vi "Instrument System Definition Example.vi"(10 "Instrument Addon Config Datalog Path":path, 11 "SysDef Path":path) -> (0 "error out":errorcluster)   [LabVIEW 2019]
uses:
  NationalInstruments.VeriStand.SystemDefinitionAPI
  Instrument System Definition API.lvlib
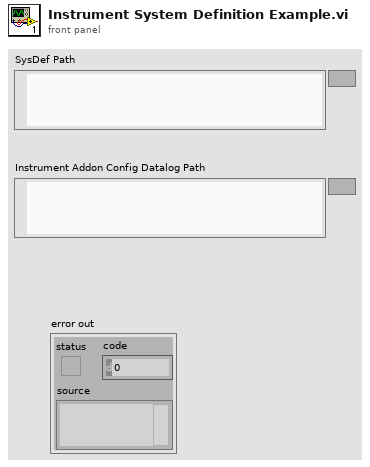
[diagram p1: front panel]
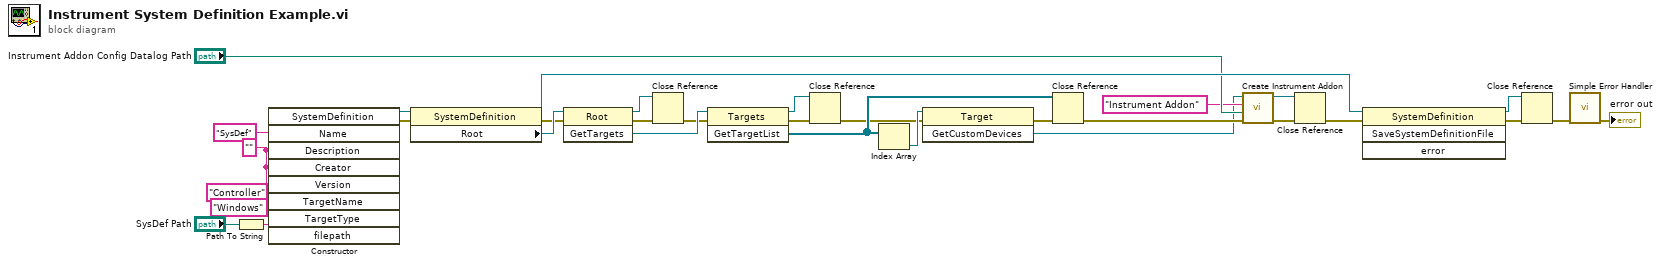
[diagram p0: block diagram]
diagram:
  w7 = "" ("Name")
  n1 = Path To String(path="SysDef Path") -> (string=w10:string)
  n2 = constructor class="SystemDefinition"("Name"="SysDef", "Description"=w7, "Creator"=w7, "Version"=w7, "TargetName"="Controller", "TargetType"="Windows", "filepath"=w10) -> (reference out=w32:refnum<k24>, error out=w28:errorcluster)  [unwired: 3 in, 8 out]
  n3 = property class="SystemDefinition"(reference=w32, error in=w28) -> (reference out=w26:refnum<k24>, error out=w27:errorcluster, "Root"=w31:refnum<k24>)
  n4 = invoke class="Root" method="GetTargets"(reference=w31, error in=w27) -> (reference out=w12:refnum<k24>, error out=w14:errorcluster, "GetTargets"=w30:refnum<k24>)  [unwired: 1 in]
  n5 = Close Reference(reference=w12, error in (no error)=w14) -> (error out=w13:errorcluster)
  n6 = invoke class="Targets" method="GetTargetList"(reference=w30, error in=w13) -> (reference out=w15:refnum<k24>, error out=w17:errorcluster, "GetTargetList"=w18:refnum<k24>[])  [unwired: 1 in]
  n7 = Close Reference(reference=w15, error in (no error)=w17) -> (error out=w16:errorcluster)
  n8 = Index Array(array=w18) -> (element=w29:refnum<k24>)  [unwired: 1 in]
  n9 = invoke class="Target" method="GetCustomDevices"(reference=w29, error in=w16) -> (error out=w20:errorcluster, "GetCustomDevices"=w3:refnum<k24>)  [unwired: 1 in, 1 out]
  n10 = Close Reference(reference=w18, error in (no error)=w20) -> (error out=w19:errorcluster)
  n11 = call "Create Instrument Addon.vi"("error in (no error)"=w19, "CD Config Path (.dat)"="Instrument Addon Config Datalog Path", "Name"="Instrument Addon", "Custom Devices Ref"=w3) -> ("error out"=w2:errorcluster, "Custom Devices Ref"=w21:refnum<k24>)  [unwired: 6 in]
  n12 = Close Reference(reference=w21, error in (no error)=w2) -> (error out=w22:errorcluster)
  n13 = invoke class="SystemDefinition" method="SaveSystemDefinitionFile"(reference=w26, error in=w22) -> (reference out=w23:refnum<k24>, error out=w24:errorcluster)  [unwired: 2 in, 2 out]
  n14 = Close Reference(reference=w23, error in (no error)=w24) -> (error out=w11:errorcluster)
  n15 = call <vilib>:"Simple Error Handler.vi"("error in (no error)"=w11) -> ("error out"=→"error out":errorcluster)  [unwired: 4 in, 4 out]
